vi "Set Control Properties.vi"(8 "error in (no error)":errorcluster, 10 "Owning VI":refnum<vi>, 11 "Control in":refnum<class "Control.lvclass">) -> (0 "error out":errorcluster, 2 "dup Owning VI":refnum<vi>, 3 "Control out":refnum<class "Control.lvclass">)   [LabVIEW 2020, in "VI Properties Editor.lvlib" / "Control.lvclass"]
doc: "Sets the properties of <B>Control in</B> by finding the reference from the control's UID and <B>Owning VI</B>."
uses:
  Control.lvclass
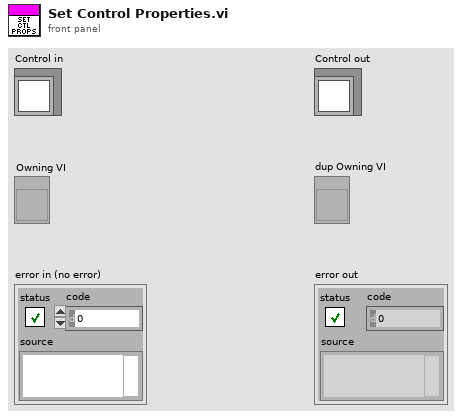
[diagram p1: front panel]
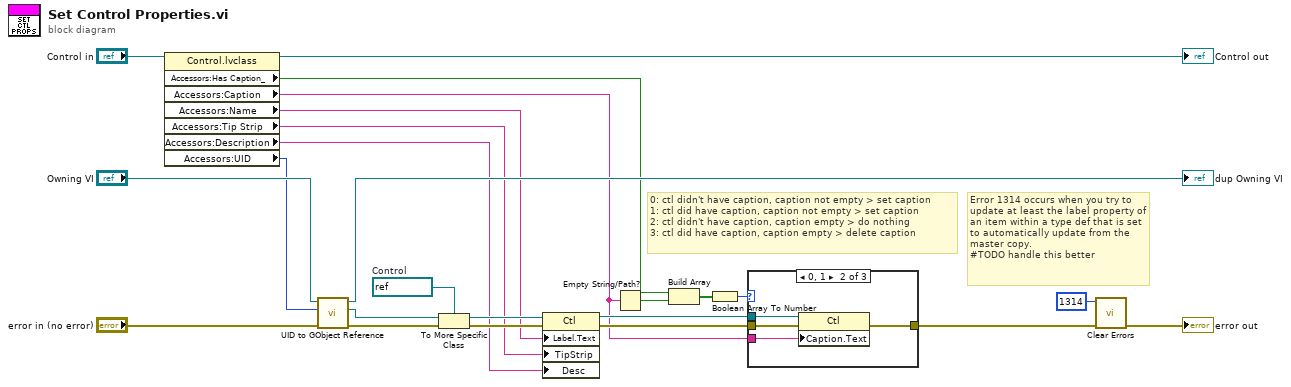
[diagram p0: block diagram]
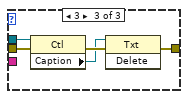
[diagram p3: hidden frame]
diagram:
  w10 = refnum<vi> refnum  # Control
  # "0: ctl didn't have caption, caption not empty > set caption\n1: ctl did have caption, caption not empty > set caption\n2: ctl didn't have caption, caption empty > do nothing\n3: ctl did have caption, caption empty > delete caption"
  # "Error 1314 occurs when you try to update at least the label property of an item within a type def that is set to automatically update from the master copy.\n#TODO handle this better"
  n1 = property class="Control.lvclass"(reference="Control in") -> (reference out=→"Control out":refnum<class "Control.lvclass">, "Accessors:Has Caption_"=w4:bool, "Accessors:Caption"=w5:string, "Accessors:Name"=w7:string, "Accessors:Tip Strip"=w18:string, "Accessors:Description"=w17:string, "Accessors:UID"=w13:i32)  [unwired: 1 in, 1 out]
  n2 = call <vilib>:"UID to GObject Reference.vi"("error in (no error)"="error in (no error)", "UID"=w13, "Owning VI"="Owning VI") -> ("error out"=w12:errorcluster, "GObject"=w11:refnum<vi>, "dup Owning VI"=→"dup Owning VI":refnum<vi>)  [unwired: 6 in]
  n3 = To More Specific Class(target class=w10, reference=w11, error in=w12) -> (specific class reference=w24:refnum<vi>, error out=w23:errorcluster)
  n4 = property class="Ctl"(reference=w24, error in=w23, "Label.Text"=w7, "TipStrip"=w18, "Desc"=w17) -> (reference out=w8:refnum<vi>, error out=w9:errorcluster)
  n5 = Empty String/Path?(string/path=w5) -> (empty?=w3:bool)
  n6 = Build Array(w4, w3) -> (w2:bool[])
  n7 = Boolean Array To Number(Boolean array=w2) -> (number=w1:u32)
  n8 = case shown="0, 1" w1 {
    tunnel: w9 -> [w25 w29 w34]
    tunnel: w8 -> [_ w28 w33]
    tunnel: w5 -> [_ w27 _]
    tunnel: [w25 w26 w31] -> w6
    frame 2, Default {
    }
    frame 0, 1 {
      n9 = property class="Ctl"(reference=w28, error in=w29, "Caption.Text"=w27) -> (error out=w26:errorcluster)  [unwired: 1 out]
    }
    frame 3 {
      n10 = property class="Ctl"(reference=w33, error in=w34) -> (error out=w32:errorcluster, "Caption"=w30:refnum<vi>)  [unwired: 1 out]
      n11 = invoke class="Txt" method="Delete"(reference=w30, error in=w32) -> (error out=w31:errorcluster)  [unwired: 1 in, 2 out]
    }
  }
  n12 = call <vilib>:"Clear Errors.vi"("error in (no error)"=w6, "specific error code to clear (0: all)"=1314) -> ("error out"=→"error out":errorcluster)  [unwired: 4 in, 1 out]
